vi "NodosPropiedad.vi"() -> ()   [LabVIEW 2020]
panel:
  in  "History Data":dbl[](array[numeric])
  out "Waveform Chart":dbl(graph)
  out "Boolean":bool
  in  "Deshabilitar":bool
  out "Cadena caracteres":string
  in  "Posición horizontal":dbl(slide) scale=0.0..400.0
  in  "Posición vertical":dbl(slide) scale=0.0..300.0
  in  "Limite":dbl
  in  "stop":bool
  out "Tank":dbl(slide) scale=0.0..10.0
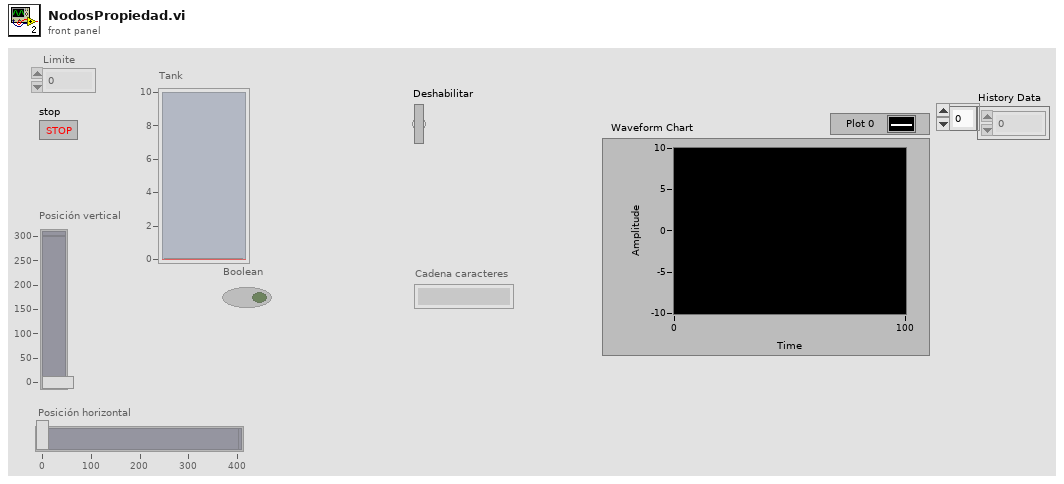
[diagram p1: front panel]
types:
  T1 = cluster{"Posición vertical":dbl, "Posición horizontal":dbl}
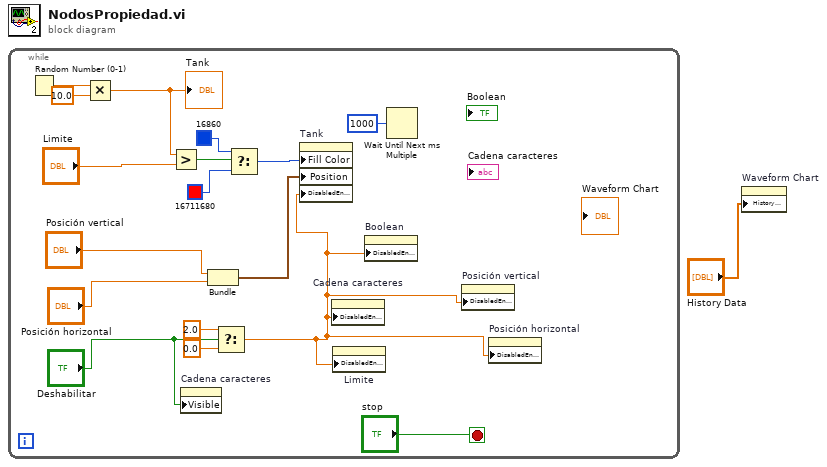
[diagram p0: block diagram]
diagram:
  n1 = while {
    stop <- "stop" stop-if-true
    n2 = Random Number (0-1)() -> (number: 0 to 1=w17:dbl)
    n3 = Multiply(x=w17, y=10.0) -> (x*y=w14:dbl)
    "Tank" <- w14
    n4 = Greater?(x=w14, y="Limite") -> (0:w13:bool)
    n5 = property on="Cadena caracteres" class="Str"("Visible"="Deshabilitar") -> ()  [unwired: 2 in, 2 out]
    n6 = Bundle "Bundle"("Posición vertical"="Posición vertical", "Posición horizontal"="Posición horizontal") -> (w6:T1)  [unwired: 1 in]
    n7 = Select(t=2.0, s="Deshabilitar", f=0.0) -> (s? t:f=w3:dbl)
    n8 = Select(t=u32 16860, s=w13, f=u32 16711680) -> (s? t:f=w9:u32)
    n9 = property on="Tank" class="Slide (strict)"("Fill Color"=w9, "Position"=w6, "DisabledEnum"=w3) -> ()  [unwired: 2 in, 2 out]
    n10 = property on="Cadena caracteres" class="Str"("DisabledEnum"=w3) -> ()  [unwired: 2 in, 2 out]
    n11 = property on="Limite" class="DigNum (strict)"("DisabledEnum"=w3) -> ()  [unwired: 2 in, 2 out]
    n12 = property on="Boolean" class="Bool (strict)"("DisabledEnum"=w3) -> ()  [unwired: 2 in, 2 out]
    n13 = Wait Until Next ms Multiple(millisecond multiple=u32 1000) -> ()  [unwired: 1 out]
    n14 = property on="Posición vertical" class="Slide (strict)"("DisabledEnum"=w3) -> ()  [unwired: 2 in, 2 out]
    n15 = property on="Posición horizontal" class="Slide (strict)"("DisabledEnum"=w3) -> ()  [unwired: 2 in, 2 out]
  }
  n16 = property on="Waveform Chart" class="WFChart (strict)"("History Data"="History Data") -> ()  [unwired: 2 in, 2 out]
